vi "PH_Beamline.get Switch State.vi"(0 "i ref in":refnum<vi>, 2 "Switch Instance":T1="PA_CH1_BB", 5 "error in (no error)":errorcluster) -> (14 "i ref out":refnum<vi>, 15 "off/false/out?":bool, 16 "on/true/in?":bool, 17 "Switch State":T2 items=["no info", "off/false/out", "on/true/in", "Failure", "Alarm", "Status 1", "Status 2", "Status 3"], 18 "off/false/out or on/true/in?":bool, 19 "error out":errorcluster)   [LabVIEW 2014]
doc: "This VI gets the state of the selected Switch."
uses:
  PH_Beamline.lvlib
  CSUser/DIMServiceTools/Status.ctl
  PH_Beamline.Switch Instances.ctl
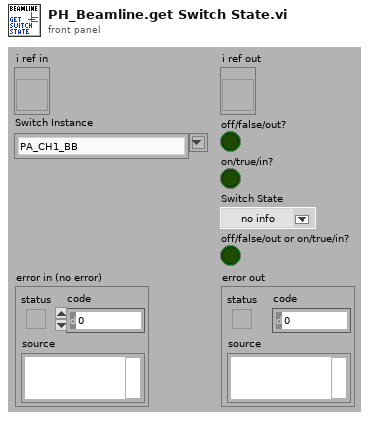
[diagram p1: front panel]
types:
  T1 = typedef "PH_Beamline.lvlib/PH_Beamline.Switch Instances.ctl" = string
  T2 = typedef "Status.ctl" = i16
  T3 = typedef "PH_Beamline.lvlib/PH_Beamline.i attribute.ctl" = cluster{"GUI Refs":cluster{"PA ok":refnum<vi>, "MA ok":refnum<vi>, "fs FE ok":refnum<vi>, "ns FE ok":refnum<vi>, "PA ED ok":refnum<vi>, "MAS ok":refnum<vi>, "Booster ok":refnum<vi>, "Mirrortower ok":refnum<vi>, "In.-Box ok":refnum<vi>, "Compressor ok":refnum<vi>, "Experiment LB ok":refnum<vi>, "Experiment LL ok":refnum<vi>, "PHELIX_Beckhoff_Watchdog":refnum<vi>, "Shutters closed":refnum<vi>, "uOPA ok":refnum<vi>, "Vacuum no shotcond Comp LB":refnum<vi>}, "Refs BL MA":refnum<vi>[], "Refs BL MA-IB":refnum<vi>[], "Refs BL fs":refnum<vi>[], "Refs BL PA ED":refnum<vi>[], "Refs BL MAS":refnum<vi>[], "Refs BL Boo":refnum<vi>[], "Refs BL ns":refnum<vi>[], "Refs BL Mirrortower":refnum<vi>[], "Refs BL Compressor":refnum<vi>[], "Refs BL Exp LB":refnum<vi>[], "Radiation Safety":cluster{"Exp Laserbay":cluster{"Ref Op Mode":refnum<vi>, "Ref Laserbay evacuated":refnum<vi>, "Tagname LB evacuated":string, "Shot Mode":T4, "Laserbay evacuated?":i32, "Tagname HV room locked":string, "HV room locked?":i32, "Ref HV room locked":refnum<vi>, "Tagname bridged?":string, "Ref Bridge":refnum<vi>, "I<1E18W/cm²":bool}, "Exp Laserlab":cluster{"Ref Op Mode":refnum<vi>, "Ref Laserlab evacuated":refnum<vi>, "Tagname LL evacuated":string, "Shot Mode":T4, "Laserlab evacuated?":i32, "Tagname bridged?":string, "Ref Bridge":refnum<vi>, "I<1E18W/cm²":bool}}, "Refs BL LL":refnum<vi>[], "PP Igni Heating GUI Refs":refnum<vi>[], "PP Igni Heating Tagnames ":string[], "Refs BL PA":cluster{"undelayed Line before Shutter":refnum<vi>[], "undelayed Line after Shutter":refnum<vi>[], "before Bypass":refnum<vi>[], "delayed Line before Shutter":refnum<vi>[], "delayed Line after Shutter":refnum<vi>[], "before Shutter Input":refnum<vi>[], "after Shutter Input":refnum<vi>[], "Bypass":refnum<vi>[], "before Shutter Exit":refnum<vi>[], "after Shutter Exit":refnum<vi>[], "to MA":refnum<vi>[], "to Lab":refnum<vi>[]}, "BL":cluster{"YLF_BL_Status":i32, "fs_BL_Status":i32, "fs_YLF_BL_Status":i32, "ns_BL_Status":i32, "PA_Input_BL_Status":i32, "PA_UnDelay_BL_Status":i32, "PA_Delay_BL_Status":i32, "PA_BL_Status":i32, "PA_Bypass_BL_Status":i32, "PA_Exit_BL_Status":i32, "PA_LL_BL_Status":i32, "LL_BL_Status":i32, "PA_MA_BL_Status":i32, "MA_Exit_BL_Status":i32, "MA_Z6_BL_Status":i32, "Z6_BL_Status":i32, "MA_LB_BL_Status":i32, "LB_TB2_BL_Status":i32, "PA_before_Bypass_BL_Status":i32, "LB_TB3_BL_Status":i32}, "State Subsystems":cluster{"PA":bool, "MA":bool, "ns FE":bool, "fs FE":bool, "PA ED":bool, "In.-Box":bool, "MAS":bool, "Booster":bool, "Mirrortower":bool, "Compressor":bool, "Experiment LB":bool, "Experiment LL":bool, "uOPA":bool}, "Status Subscriber Information":T5, "Refs BL uOPA":refnum<vi>[], "PA Doublepulse Mode?":bool, "Windowshutter Laserbay TB2 not relevant?":bool, "Windowshutter Laserbay TB3 not relevant?":bool, "Vacuum @ Compressor LB not relevant?":bool, "PA_Input_2_Beam_6PWpGUI not linked?":bool, "PA_Input_Delay_6PGUI not linked?":bool}
  T4 = typedef "Operation Mode.ctl" = i32
  T5 = typedef "PH_Beamline.lvlib/PH_Beamline.Status Subscriber Information.ctl" = cluster{"fs Swich YLF":T6, "fs Exit Shutter":T6, "ns Exit Shutter":T6, "PA Input Shutter":T6, "PA PC WP":T6, "PA PC WP 2":T6, "PA Bypass In":T6, "PA Bypass Out":T6, "PA CH 1":T6, "PA delayed":T6, "PA non delayed":T6, "PA Exit Shutter":T6, "PA Switch Lab":T6, "PA Bridge CH Input MA":T6, "MA Diffusor IB":T6, "MA IB Ready":T6, "MA CH 1":T6, "MA CH 2":T6, "MA CH 3":T6, "MA CH 4":T6, "MA Shutter Align Cam":T6, "MA Position MM5":T6, "Calorimeter Switch":T6, "BL Z6 CH 9":T6, "BL Z6 Beamdump":T6, "BL Z6 Shutter":T6, "COS Sensitivity Switch":T6, "Exp LB Shutter":T6, "Exp LB TB 2":T6, "Exp LB TB 3":T6, "PA LL Input CH":T6, "PA LL Output CH":T6, "LL Comp Input Shutter":T6, "LL Comp Output Shutter":T6, "LL Comp FF Shutter":T6, "Exp LL Shutter":T6, "MA IM In IB":T6, "MA IM Out IB":T6, "MA DB In IB":T6, "MA DB Out IB":T6, "Exp LB Shutter Interlock":T6, "Exp LL Shutter Interlock":T6}
  T6 = typedef "PH_BL-Master.lvlib/PH_BL-Master.Status Subscriber Information.ctl" = cluster{"Index of element":i32, "Attributeset":T7}
  T7 = typedef "PH_BL-Master.lvlib/PH_BL-Master.Attribute Set.ctl" = enum16{"Boolean Status Service Subscriber", "Picture Status Service Subscriber"}
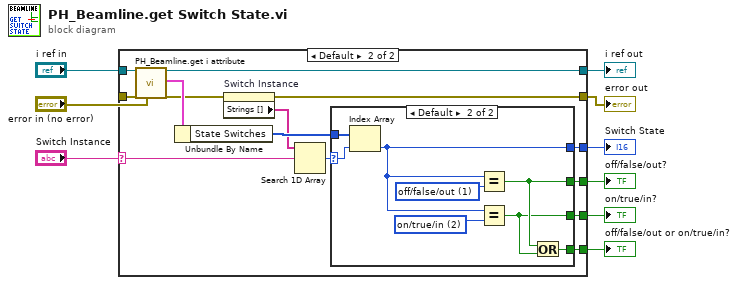
[diagram p0: block diagram]
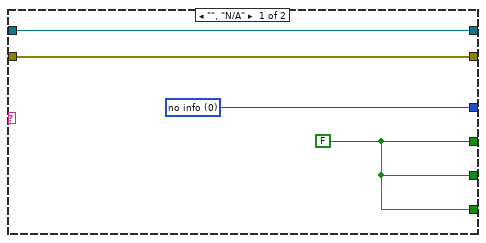
[diagram p2: hidden frame]
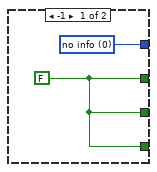
[diagram p3: hidden frame]
diagram:
  n1 = case shown="Default" "Switch Instance" {
    selector: "Switch Instance" -> [_ w19]
    tunnel: "error in (no error)" -> [w12 w26]
    tunnel: "i ref in" -> [w13 w25]
    tunnel: [w13 w24] -> w7
    tunnel: [w11 w23] -> w6
    tunnel: [w12 w20] -> w5
    tunnel: [w10 w16] -> w1
    tunnel: [w10 w15] -> w3
    tunnel: [w10 w14] -> w2
    frame "", "N/A" {
      w11 = T2 0 items=["no info", "off/false/out", "on/true/in", "Failure", "Alarm", "Status 1", "Status 2", "Status 3"] ("State")
      w10 = FALSE
    }
    frame Default {
      n2 = call "PH_Beamline.get i attribute.vi"("i ref in"=w25, "error in (no error)"=w26) -> ("i ref out"=w24:refnum<vi>, "i attribute"=w27:T3, "error out"=w21:errorcluster)  [unwired: 15 in]
      n3 = Unbundle By Name(w27) -> ("State Switches"=w22:T2[])
      n4 = property on="Switch Instance" class="CmbBox (strict)"(error in=w21) -> (error out=w20:errorcluster, "Strings []"=w17:string[])  [unwired: 1 in, 1 out]
      n5 = Search 1D Array(1D array=w17, element=w19) -> (index of element=w18:i32)  [unwired: 1 in]
      n6 = case shown="Default" w18 {
        selector: w18 -> [_ w36]
        tunnel: [w29 w34] -> w23
        tunnel: w22 -> [_ w37]
        tunnel: [w28 w32] -> w16
        tunnel: [w28 w31] -> w15
        tunnel: [w28 w30] -> w14
        frame -1 {
          w28 = FALSE
          w29 = T2 0 items=["no info", "off/false/out", "on/true/in", "Failure", "Alarm", "Status 1", "Status 2", "Status 3"] ("State")
        }
        frame Default {
          w33 = T2 2 items=["no info", "off/false/out", "on/true/in", "Failure", "Alarm", "Status 1", "Status 2", "Status 3"] ("y")
          w35 = T2 1 items=["no info", "off/false/out", "on/true/in", "Failure", "Alarm", "Status 1", "Status 2", "Status 3"] ("y")
          n7 = Index Array(array=w37, index=w36) -> (element=w34:T2)
          n8 = Equal?(x=w34, y=w35) -> (x = y?=w32:bool)
          n9 = Equal?(x=w34, y=w33) -> (x = y?=w31:bool)
          n10 = Or(x=w32, y=w31) -> (x .or. y?=w30:bool)
        }
      }
    }
  }
  "i ref out" <- w7
  "error out" <- w5
  "Switch State" <- w6
  "off/false/out?" <- w1
  "on/true/in?" <- w3
  "off/false/out or on/true/in?" <- w2
